vi "Intake Logic.vi"(1 "Intake Info In":T2) -> (0 "Intake Info Out":T2)   [LabVIEW 2013]
uses:
  <vilib>/Rock Robotics/WPI/Solenoid/WPI_SolenoidValue.ctl
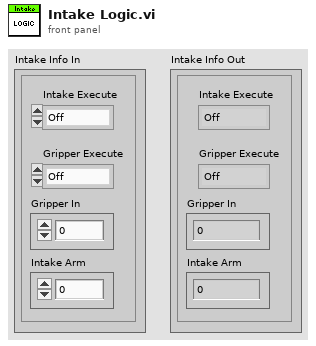
[diagram p1: front panel]
types:
  T1 = typedef "WPI_SolenoidValue.ctl" = enum16{"Off", "On", "Forward", "Reverse"}
  T2 = cluster{"Intake Execute":T1, "Gripper Execute":T1, "Gripper In":dbl, "Intake Arm":dbl}
  T3 = typedef "WPI_RelayValue.ctl" = enum16{"Off", "On", "Forward", "Reverse"}
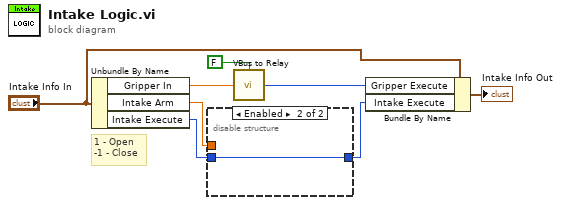
[diagram p0: block diagram]
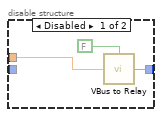
[diagram p2: hidden frame]
diagram:
  # "1 - Open\n-1 - Close"
  n1 = Unbundle By Name("Intake Info In") -> ("Gripper In"=w6:dbl, "Intake Arm"=w3:dbl, "Intake Execute"=w1:T1)
  n2 = disable-structure shown="Enabled" {
    disable-tunnel: w3 -> [w10 _]
    disable-tunnel: [w9 w12] -> w2
    disable-tunnel: w1 -> [_ w12]
    frame Disabled {
      n3 = call "VBus to Relay.vi"("Invert Relay? (F)"=FALSE, "Motor VBus"=w10) -> ("RelayValue"=w9:T3)  [unwired: 2 in]
    }
    frame Enabled {
    }
  }
  n4 = call "VBus to Relay.vi"("Invert Relay? (F)"=FALSE, "Motor VBus"=w6) -> ("RelayValue"=w4:T3)  [unwired: 2 in]
  n5 = Bundle By Name(cluster="Intake Info In", "Gripper Execute"=w4, "Intake Execute"=w2) -> (→"Intake Info Out":T2)
